vi "Read Test Tree reference.vi"(8 "error in (no error)":errorcluster, 11 "Test Tree in":refnum<class "Test Tree.lvclass">) -> (0 "error out":errorcluster, 2 "Test Tree reference":refnum<vi>, 3 "Test Tree out":refnum<class "Test Tree.lvclass">)   [LabVIEW 2020, in "Test Tree.lvclass"]
uses:
  Test Tree.lvclass
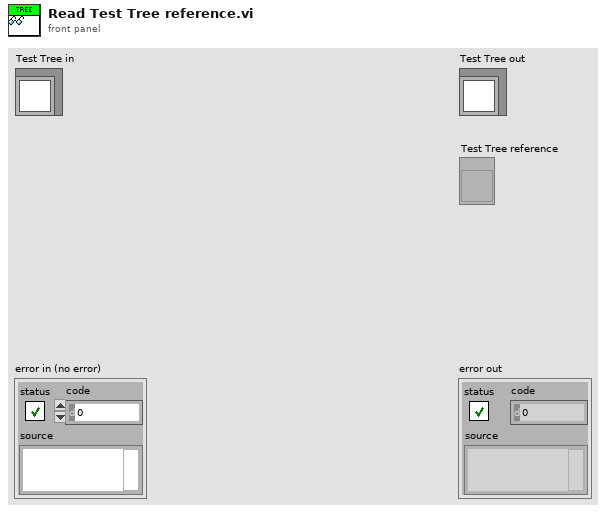
[diagram p1: front panel]
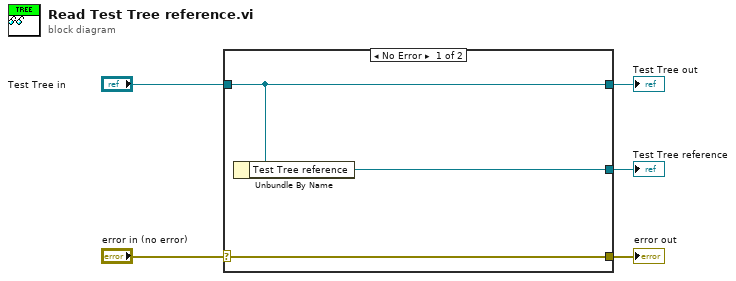
[diagram p0: block diagram]
diagram:
  n1 = case shown="No Error" "error in (no error)" {
    selector: "error in (no error)" -> [w8 w9]
    tunnel: [w8 w9] -> w4
    tunnel: [w7 w10] -> w2
    tunnel: "Test Tree in" -> [w7 w10]
    tunnel: [w6 _] -> w1
    frame No Error {
      n2 = Unbundle By Name(w7) -> ("Test Tree reference"=w6:refnum<vi>)
    }
    frame Error {
    }
  }
  "error out" <- w4
  "Test Tree out" <- w2
  "Test Tree reference" <- w1
